vi "Test_Register Dummy Service.vi"   [LabVIEW 2020]
uses:
  <vilib>/TAF/Discovery Client/RPC Messages/NIMeasurementServices_RegisterServiceRequest.ctl
  <vilib>/TAF/Discovery Client/RPC Messages/NIMeasurementServices_ServiceDescriptor.ctl
  <vilib>/TAF/Discovery Client/RPC Messages/NIMeasurementServices_ServiceLocation.ctl
  <vilib>/TAF/Discovery Client/Discovery_client.lvlib
types:
  T1 = typedef "gprc-lvsupport-release.lvlib/grpcId.ctl" = u64
  T2 = typedef "Discovery_client.lvlib/NIMeasurementServices_RegisterServiceRequest.ctl" = cluster{"service_description":T3, "provided_services":string[], "location":T4}
  T3 = typedef "Discovery_client.lvlib/NIMeasurementServices_ServiceDescriptor.ctl" = cluster{"service_id":string, "name":string, "description_url":string, "service_class":string}
  T4 = typedef "Discovery_client.lvlib/NIMeasurementServices_ServiceLocation.ctl" = cluster{"location":string, "optimal_route":string, "insecure_port":string, "ssl_authenticated_port":string}
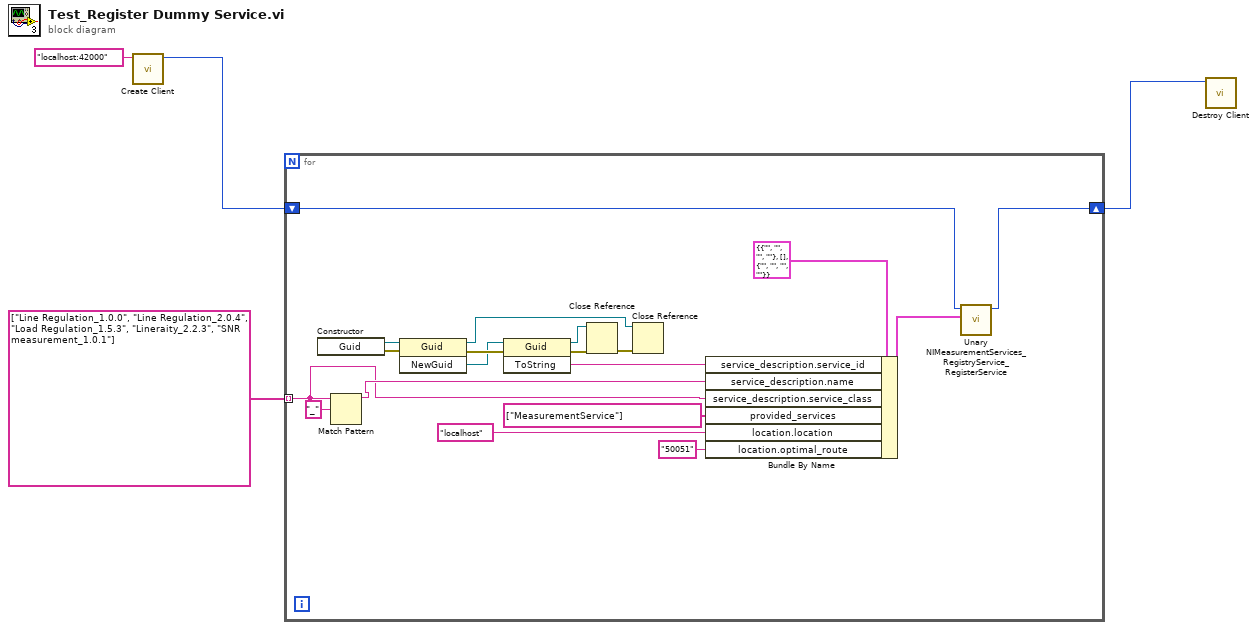
[diagram p0: block diagram]
diagram:
  n1 = call <vilib>:"Create Client.vi"("address"="localhost:42000") -> ("gRPC ID Out"=w3:T1)  [unwired: 9 in, 1 out]
  n2 = for {
    shift-right: [w14] -> w2
    shift-left: w3 -> [w15]
    tunnel: string[] ["Line Regulation_1.0.0", "Line Regulation_2.0.4", "Load Regulation_1.5.3", "Lineraity_2.2.3", "SNR measurement_1.0.1"] -> [w6] mode=indexing
    n3 = constructor class="Guid"() -> (reference out=w17:refnum<k24>, error out=w16:errorcluster)  [unwired: 3 in, 1 out]
    n4 = Match Pattern(string=w6, regular expression="_") -> (before substring=w7:string)  [unwired: 1 in, 3 out]
    n5 = invoke class="Guid" method="NewGuid"(reference=w17, error in=w16) -> (reference out=w23:refnum<k24>, error out=w20:errorcluster, "NewGuid"=w18:refnum<k24>)  [unwired: 1 in]
    n6 = invoke class="Guid" method="ToString"(reference=w18, error in=w20) -> (reference out=w21:refnum<k24>, error out=w19:errorcluster, "ToString"=w13:string)  [unwired: 1 in]
    n7 = Close Reference(reference=w21, error in (no error)=w19) -> (error out=w22:errorcluster)
    n8 = Close Reference(reference=w23, error in (no error)=w22) -> ()  [unwired: 1 out]
    n9 = Bundle By Name(cluster=T2 {"service_description"={"service_id"="", "name"="", "description_url"="", "service_class"=""}, "provided_services"=[], "location"={"location"="", "optimal_route"="", "insecure_port"="", "ssl_authenticated_port"=""}} ("Request Data"), "service_description.service_id"=w13, "service_description.name"=w7, "service_description.service_class"=w6, "provided_services"=string[] ["MeasurementService"], "location.location"="localhost", "location.optimal_route"="50051") -> (w12:T2)
    n10 = call <vilib>:"Unary NIMeasurementServices_RegistryService_RegisterService.vi"("Request Data"=w12, "gRPC ID"=w15) -> ("gRPC ID out"=w14:T1)  [unwired: 7 in, 2 out]
  }
  n11 = call <vilib>:"Destroy Client.vi"("gRPC ID"=w2) -> ()  [unwired: 10 in, 1 out]
